vi "attribute_cache_read.vi"(7 "Attribute":T1={"Identifier"="", "Descriptive Name"="", "Data Type"=enum."Integer 32", "Command"="", "Access"=enum."Read/Write", "Range Table"="", "Read Callback"="", "Write Callback"="", "Supported Models"="", "Instrument Options"="", "Index"=0, "OPC Wait"=FALSE, "No Status Check"=FALSE, "Cache Only"=FALSE}, 8 "error in":errorcluster caption="error in (no error)", 9 "Direct Attribute ID (Attribute cluster)":string, 11 "VISA resource name":refnum<visa-resource-name>) -> (0 "error out":errorcluster, 1 "Int32 out":i32, 2 "Double out":dbl, 3 "VISA resource name out":refnum<visa-resource-name>, 4 "String out":string, 5 "Int64 out":i64, 6 "Boolean out":bool, 10 "Exists in cache":bool)   [LabVIEW 2020, in "Rohde&Schwarz RTx Oscilloscopes.lvlib" / "rsidr_core.lvlib"]
uses:
  rsidr_core.lvlib
  type_Attribute.ctl
  type_Attribute_Data_Type.ctl
  type_ReadWriteAccess.ctl
  _type_Operation_Fgv_Cache.ctl
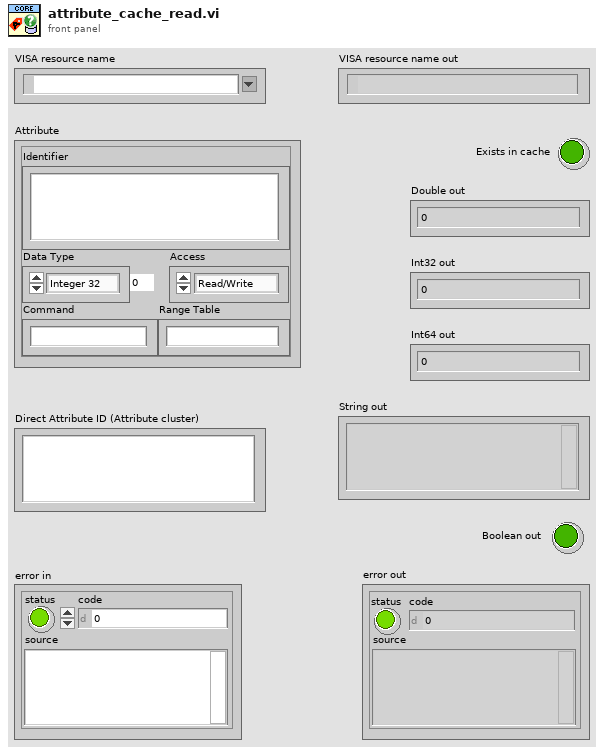
[diagram p1: front panel]
types:
  T1 = typedef "Rohde&Schwarz RTx Oscilloscopes.lvlib/rsidr_core.lvlib/type_Attribute.ctl" = cluster{"Identifier":string, "Descriptive Name":string, "Data Type":T2, "Command":string, "Access":T3, "Range Table":string, "Read Callback":string, "Write Callback":string, "Supported Models":string, "Instrument Options":string, "Index":i32, "OPC Wait":bool, "No Status Check":bool, "Cache Only":bool}
  T2 = typedef "Rohde&Schwarz RTx Oscilloscopes.lvlib/rsidr_core.lvlib/type_Attribute_Data_Type.ctl" = enum16{"Integer 32", "Double", "String", "Boolean", "None", "Integer 64", "RawString"}
  T3 = typedef "Rohde&Schwarz RTx Oscilloscopes.lvlib/rsidr_core.lvlib/type_ReadWriteAccess.ctl" = enum16{"Read Only", "Write Only", "Read/Write"}
  T4 = typedef "Rohde&Schwarz RTx Oscilloscopes.lvlib/rsidr_core.lvlib/_type_Operation_Fgv_Cache.ctl" = enum16{"Initialize", "Get Cached Value", "Set Cached Value", "Clear"}
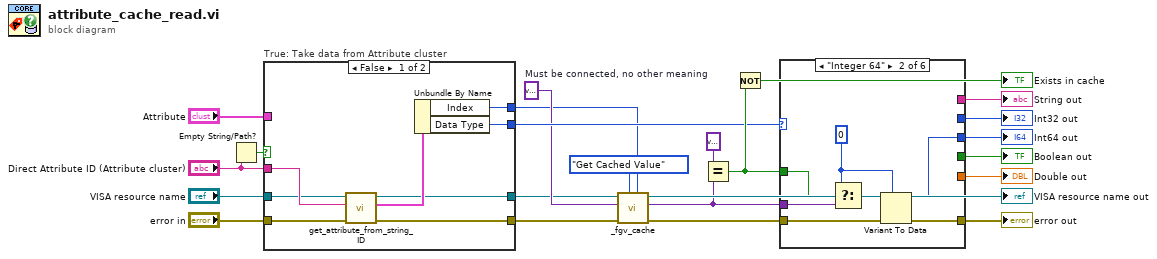
[diagram p0: block diagram]
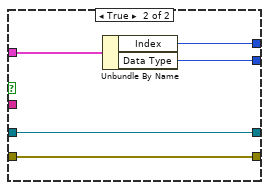
[diagram p2: hidden frame]
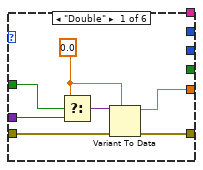
[diagram p3: hidden frame]
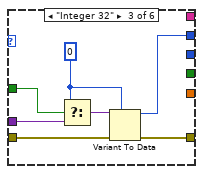
[diagram p4: hidden frame]
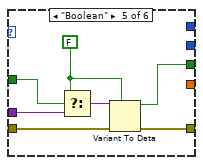
[diagram p6: hidden frame]
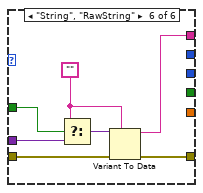
[diagram p7: hidden frame]
diagram:
  w4 = variant  # Must be connected, no other meaning
  n1 = Empty String/Path?(string/path="Direct Attribute ID (Attribute cluster)") -> (empty?=w10:bool)
  n2 = case "True: Take data from Attribute cluster" shown="False" w10 {
    tunnel: "Direct Attribute ID (Attribute cluster)" -> [w29 _]
    tunnel: "error in" -> [w31 w33]
    tunnel: [w30 w33] -> w7
    tunnel: "Attribute" -> [_ w36]
    tunnel: [w28 w35] -> w3
    tunnel: [w27 w34] -> w5
    tunnel: "VISA resource name" -> [w25 w32]
    tunnel: [w24 w32] -> w1
    frame False {
      n3 = call "get_attribute_from_string_ID.vi"("error in"=w31, "Attribute ID in"=w29, "VISA resource name"=w25) -> ("error out"=w30:errorcluster, "Attribute out"=w26:T1, "VISA resource name out"=w24:refnum<visa-resource-name>)  [unwired: 6 in]
      n4 = Unbundle By Name(w26) -> ("Index"=w28:i32, "Data Type"=w27:T2)
    }
    frame True {
      n5 = Unbundle By Name(w36) -> ("Index"=w35:i32, "Data Type"=w34:T2)
    }
  }
  n6 = call "_fgv_cache.vi"("Index in"=w3, "Operation"=_type_Operation_Fgv_Cache."Get Cached Value" ("Operation (1: Get Cached Value)"), "error in"=w7, "Value in"=w4, "VISA resource name"=w1) -> ("error out"=w22:errorcluster, "Cache Value out"=w17:variant, "VISA resource name out"=→"VISA resource name out":refnum<visa-resource-name>)  [unwired: 4 in]
  n7 = Equal?(x=variant ("Value"), y=w17) -> (x = y?=w16:bool)
  n8 = Not(x=w16) -> (.not. x?=→"Exists in cache":bool)
  n9 = case shown="\"Integer 64\"" w5 {
    tunnel: w17 -> [w39 w46 w53 _ w61 w68]
    tunnel: w22 -> [w41 w48 w55 w58 w63 w70]
    tunnel: [w40 w47 w54 w58 w62 w69] -> w20
    tunnel: [w38 _ _ _ _ _] -> w21
    tunnel: w16 -> [w37 w45 w52 _ w60 w67]
    tunnel: [_ _ _ _ w59 _] -> w15
    tunnel: [_ _ _ _ _ w66] -> w14
    tunnel: [_ w44 _ _ _ _] -> w13
    tunnel: [_ _ w51 _ _ _] -> w12
    frame "Double" {
      w43 = 0.0 ("type")
      n10 = Select(t=w43, s=w37, f=w39) -> (s? t:f=w42:variant)
      n11 = Variant To Data(error in=w41, type=w43, Variant=w42) -> (data=w38:dbl, error out=w40:errorcluster)
    }
    frame "Integer 64" {
      w50 = i64 0 ("type")
      n12 = Select(t=w50, s=w45, f=w46) -> (s? t:f=w49:variant)
      n13 = Variant To Data(error in=w48, type=w50, Variant=w49) -> (data=w44:i64, error out=w47:errorcluster)
    }
    frame "Integer 32" {
      w57 = 0 ("type")
      n14 = Select(t=w57, s=w52, f=w53) -> (s? t:f=w56:variant)
      n15 = Variant To Data(error in=w55, type=w57, Variant=w56) -> (data=w51:i32, error out=w54:errorcluster)
    }
    frame "None" {
    }
    frame "Boolean" {
      w65 = FALSE
      n16 = Select(t=w65, s=w60, f=w61) -> (s? t:f=w64:variant)
      n17 = Variant To Data(error in=w63, type=w65, Variant=w64) -> (data=w59:bool, error out=w62:errorcluster)
    }
    frame "String", "RawString" {
      w72 = "" ("type")
      n18 = Select(t=w72, s=w67, f=w68) -> (s? t:f=w71:variant)
      n19 = Variant To Data(error in=w70, type=w72, Variant=w71) -> (data=w66:string, error out=w69:errorcluster)
    }
  }
  "error out" <- w20
  "Double out" <- w21
  "Int64 out" <- w13
  "Int32 out" <- w12
  "String out" <- w14
  "Boolean out" <- w15
